vi "Convert HSL to RGB.vi"(9 "L (%)":dbl, 10 "S (%)":dbl, 11 "H (deg)":dbl format="%#_2p") -> (3 "Color Box":u32(colorbox)=16777215)   [LabVIEW 2015, in "ColorSelector.lvclass"]
doc: "This VI will convert the HSL Color Scale to the RGB Color Scale.\n<b> </b> <b> </b>\n©2017 Q Software Innovations, LLC (QSI)\nwritten by Quentin Alldredge\nproduced in LabVIEW 2015\n\nsupport@qsoftwareinnovations.com\nwww.qsoftwareinnovations.com\n\nAll rights reserved.\n\nRedistribution and use in source and binary forms, with or without modification, are permitted provided that the following conditions are met:\n\n * Redistributions of source code must retain the above copyright notice, this list of conditions and the following disclaimer.\n * Redistributions in binary form must reproduce the above copyright notice, this list of conditions and the following disclaimer in the documentation and/or other materials provided with the distribution.\n * Neither the name of Q Software Innovations, LLC. nor the names of its contributors may be used to endorse or promote products derived from this software without specific prior written permission.\n\nTHIS SOFTWARE IS PROVIDED BY THE COPYRIGHT HOLDERS AND CONTRIBUTORS \"AS IS\" AND ANY EXPRESS OR IMPLIED WARRANTIES, INCLUDING, BUT NOT LIMITED TO, THE IMPLIED WARRANTIES OF MERCHANTABILITY AND FITNESS FOR A PARTICULAR PURPOSE ARE DISCLAIMED. IN NO EVENT SHALL THE COPYRIGHT OWNER OR CONTRIBUTORS BE LIABLE FOR ANY DIRECT, INDIRECT, INCIDENTAL, SPECIAL, EXEMPLARY, OR CONSEQUENTIAL DAMAGES (INCLUDING, BUT NOT LIMITED TO, PROCUREMENT OF SUBSTITUTE GOODS OR SERVICES; LOSS OF USE, DATA, OR PROFITS; OR BUSINESS INTERRUPTION) HOWEVER CAUSED AND ON ANY THEORY OF LIABILITY, WHETHER IN CONTRACT, STRICT LIABILITY, OR TORT (INCLUDING NEGLIGENCE OR OTHERWISE) ARISING IN ANY WAY OUT OF THE USE OF THIS SOFTWARE, EVEN IF ADVISED OF THE POSSIBILITY OF SUCH DAMAGE."
uses:
  ColorSelector.lvclass
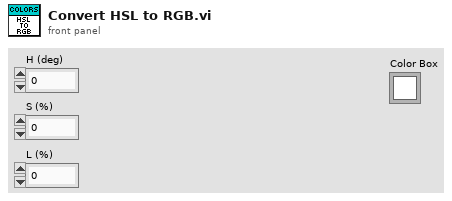
[diagram p1: front panel]
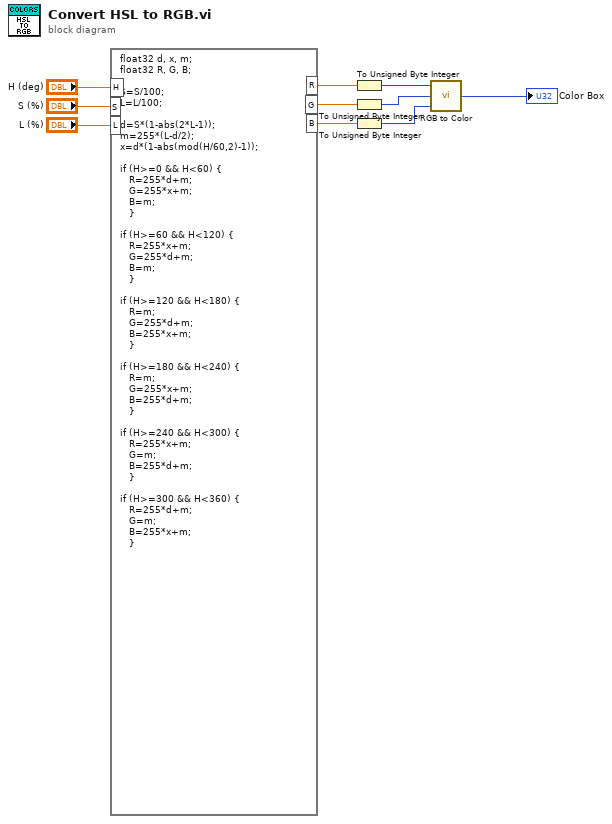
[diagram p0: block diagram]
diagram:
  n1 = formula code="float32 d, x, m;\nfloat32 R, G, B;\n\nS=S/100;\nL=L/100;\n\nd=S*(1-abs(2*L-1));\nm=255*(L-d/2);\nx=d*(1-abs(mod(H/60,2)-1));\n\nif (H>=0 && H<60) {\n   R=255*d+m;\n   G=255*x+m;\n   B=m;\n   }\n\nif (H>=60 && H<120) {\n   R=255*x+m;\n   G=255*d+m;\n   B=m;\n   }\n\nif (H>=120 && H<180) {\n   R=m;\n   G=255*d+m;\n   B=255*x+m;\n   }\n\nif (H>=180 && H<240) {\n   R=m;\n   G=255*x+m;\n   B=255*d+m;\n   }\n\nif (H>=240 && H<300) {\n   R=255*x+m;\n   G=m;\n   B=255*d+m;\n   }\n\nif (H>=300 && H<360) {\n   R=255*d+m;\n   G=m;\n   B=255*x+m;\n   }"("H"="H (deg)", "S"="S (%)", "L"="L (%)") -> ("R"=w3:sgl, "G"=w2:sgl, "B"=w1:sgl)
  n2 = To Unsigned Byte Integer(number=w3) -> (unsigned 8bit integer=w5:u8)
  n3 = To Unsigned Byte Integer(number=w2) -> (unsigned 8bit integer=w6:u8)
  n4 = To Unsigned Byte Integer(number=w1) -> (unsigned 8bit integer=w7:u8)
  n5 = call <vilib>:"RGB to Color.vi"("B"=w7, "G"=w6, "R"=w5) -> ("Color"=→"Color Box":u32)
